vi "download_calibration.vi"(6 "configuration":u64, 9 "port":u16, 10 "host":string, 11 "path in":path=path "hl2ss_ulm.dll") -> (0 "calibration":u64, 1 "port":u16, 2 "host":string, 3 "path out":path, 4 "configuration":u64, 5 "calibration_handle":u64)   [LabVIEW 2023]
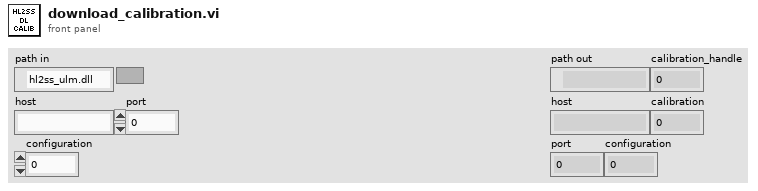
[diagram p1: front panel]
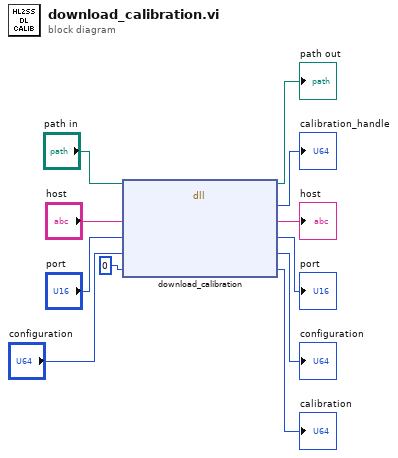
[diagram p0: block diagram]
diagram:
  n1 = dll-call lib="C:/Users/jcds/Documents/GitHub/hl2ss/extensions/client_labview/hl2ss_ulm.dll" fn="download_calibration"(path in="path in", "host"="host", "port"="port", "configuration"="configuration", "calibration"=u64 0) -> (path out=→"path out":path, "return type"=→"calibration_handle":u64, "host"=→"host":string, "port"=→"port":u16, "configuration"=→"configuration":u64, "calibration"=→"calibration":u64)  [unwired: 2 in, 1 out]
